vi "PH_Sequencer.check for PA Defocus.vi"(1 "Heads":T1[](array[typedef])) -> (0 "PA Defocus must be set?":bool)   [LabVIEW 2014, in "PH_Sequencer.lvlib"]
uses:
  PH_Sequencer.lvlib
  PH_BeamlineInformation/PH_BeamlineInformation.Head.ctl
  PH_PP_Common/PH_PP_Common.PUs.ctl
  PH_BeamlineInformation/PH_BeamlineInformation.lvlib
  PH_PP_Common/PH_PP_Common.lvlib
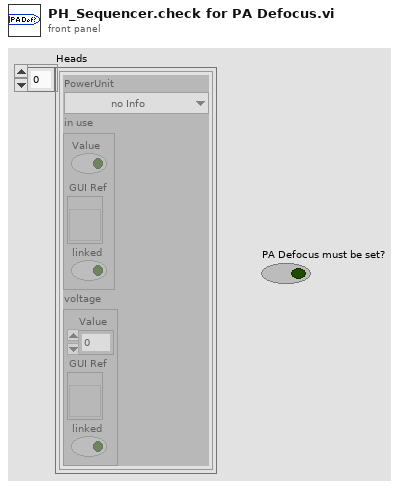
[diagram p1: front panel]
types:
  T1 = typedef "PH_BeamlineInformation.lvlib/PH_BeamlineInformation.Head.ctl" = cluster{"PowerUnit":T2, "in use":cluster{"Value":bool, "GUI Ref":refnum<vi>, "linked":bool}, "voltage":cluster{"Value":dbl, "GUI Ref":refnum<vi>, "linked":bool}}
  T2 = typedef "PH_PP_Common.lvlib/PH_PP_Common.PUs.ctl" = enum16{"no Info", "PA-19mm-1", "PA-19mm-2", "PA-45mm-PILC", "PA-45mm-MAIN", "MA-PU-1", "MA-PU-2", "MA-PU-3", "MA-PU-4", "MA-PU-5", "MA-PU-6", "MA-FR", "MA-PILC", "PA-45mm-DP"}
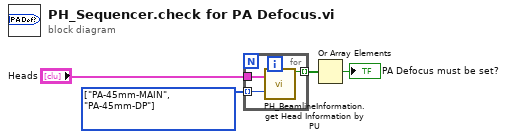
[diagram p0: block diagram]
diagram:
  w1 = T2[] [enum."PA-45mm-MAIN", enum."PA-45mm-DP"] items=["no Info", "PA-19mm-1", "PA-19mm-2", "PA-45mm-PILC", "PA-45mm-MAIN", "MA-PU-1", "MA-PU-2", "MA-PU-3", "MA-PU-4", "MA-PU-5", "MA-PU-6", "MA-FR", "MA-PILC", "PA-45mm-DP"]
  n1 = for {
    tunnel: "Heads" -> [w7]
    tunnel: w1 -> [w6] mode=indexing
    tunnel: [w5] -> w3 mode=indexing
    n2 = call "PH_BeamlineInformation.get Head Information by PU.vi"("Heads"=w7, "Power Unit"=w6) -> ("In Use?"=w5:bool)  [unwired: 12 in, 5 out]
  }
  n3 = Or Array Elements(Boolean array=w3) -> (logical OR=→"PA Defocus must be set?":bool)
